vi "__Alicat SD_Test.vi"() -> ()   [LabVIEW 2017]
uses:
  __Alicat SD_ReadingCluster.ctl
  __Alicat SD_Hardware_Module.ctl
panel:
  in  "Used ?":bool=TRUE
  out "Timeout":bool
  in  "CambiarAdd":bool
  out "ParsedReading":T1={"ID"="", "Pressure"=13.55, "Temperature"=28.56, "Volumetric"=-1.9, "Mass"=-1.7, "SetPoint"=250.0, "Gas"=""} {"SetPoint" format="%.2f"; "Mass" format="%.2f"; "Volumetric" format="%.2f"; "Temperature" format="%.2f"; "Pressure" format="%.2f"}
  out "SetPoint (64000=FullScale)":i32=32000 min=0 max=64000 step=1
  in  "Address":string="A"
  out "Cycle":i32
  out "error out":errorcluster
  in  "SetFlow":bool
  in  "VISA resource name":refnum<visa-resource-name>
  in  "stop":bool
  # "Alicat mfc test routine"
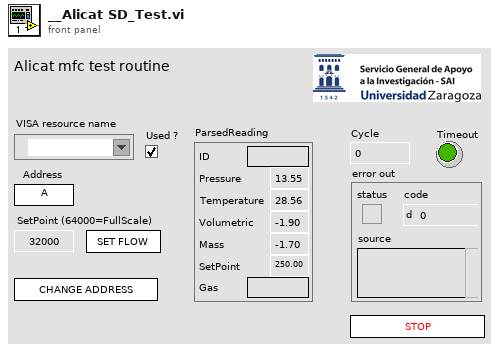
[diagram p1: front panel]
types:
  T1 = typedef "__Alicat SD_ReadingCluster.ctl" = cluster{"ID":string, "Pressure":sgl, "Temperature":sgl, "Volumetric":sgl, "Mass":sgl, "SetPoint":sgl, "Gas":string}
  T2 = typedef "__Alicat SD_Hardware_Module.ctl" = enum16{"Initialize", "Send Setpoint", "Read Data", "Change Address", "Shutdown"}
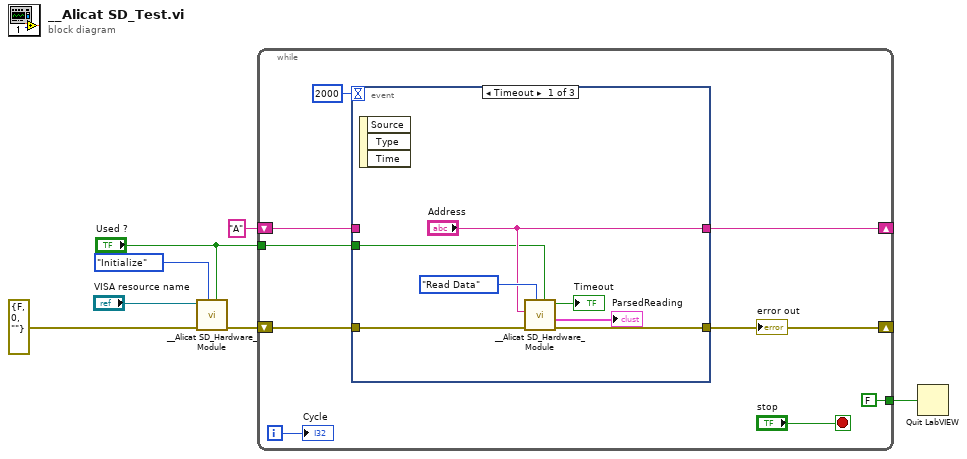
[diagram p0: block diagram]
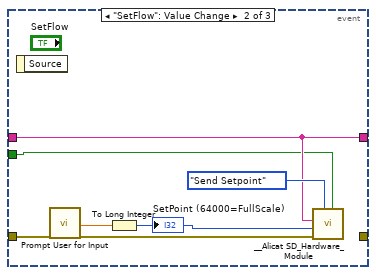
[diagram p2: hidden frame]
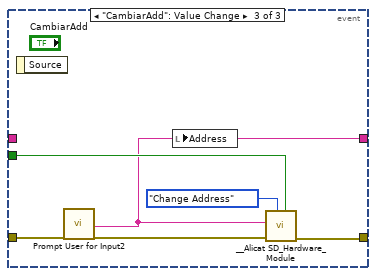
[diagram p3: hidden frame]
diagram:
  n1 = call "__Alicat SD_Hardware_Module.vi"("Used ?"="Used ?", "Command"=__Alicat_SD_Hardware_Module."Initialize", "error in (no error)"=errorcluster {"status"=FALSE, "code"=0, "source"=""}, "VISA resource name"="VISA resource name") -> ("error out"=w7:errorcluster)  [unwired: 4 in, 3 out]
  n2 = while {
    shift-right: [w12] -> _
    shift-left: w7 -> [w13]
    tunnel: [FALSE ("stop")] -> w4
    shift-right: [w10] -> _
    shift-left: "A" ("Address") -> [w11]
    tunnel: "Used ?" -> [w9]
    i -> [w16]
    stop <- "stop" stop-if-true
    n3 = event shown="[0] Timeout" {
      selector: _ -> [_ _ _]
      dyn-events: _ -> [_ _ _]
      timeout: 2000 -> [_ _ _]
      tunnel: w13 -> [w20 w28 w34]
      tunnel: [w19 _ w35] -> w12
      tunnel: w11 -> [_ w29 _]
      tunnel: ["Address" w29 w31] -> w10
      tunnel: w9 -> [w17 w24 w32]
      event Timeout {
        n4 = event-data() -> ()  [unwired: 1 in, 3 out]
        n5 = call "__Alicat SD_Hardware_Module.vi"("Used ?"=w17, "Command"=__Alicat_SD_Hardware_Module."Read Data", "error in (no error)"=w20, "Address"="Address") -> ("error out"=w19:errorcluster, "ParsedReading"=→"ParsedReading":T1, "Timeout"=→"Timeout":bool)  [unwired: 4 in, 1 out]
      }
      event "SetFlow": Value Change {
        n6 = event-data() -> ()  [unwired: 1 in, 1 out]
        n7 = call "Prompt User for Input"("error in (no error)"=w28) -> ("Setpoint"=w26:dbl, "error out"=w27:errorcluster)  [unwired: 16 in, 1 out]
        n8 = To Long Integer(number=w26) -> (32bit integer=w25:i32)
        "SetPoint (64000=FullScale)" <- w25
        n9 = call "__Alicat SD_Hardware_Module.vi"("Used ?"=w24, "Command"=__Alicat_SD_Hardware_Module."Send Setpoint", "error in (no error)"=w27, "SetPoint (64000=FullScale)"=w25, "Address"=w29) -> ()  [unwired: 3 in, 4 out]
      }
      event "CambiarAdd": Value Change {
        n10 = event-data() -> ()  [unwired: 1 in, 1 out]
        n11 = call "Prompt User for Input2"("error in (no error)"=w34) -> ("Setpoint"=w31:string, "error out"=w33:errorcluster)  [unwired: 16 in, 1 out]
        n12 = local write "Address"(w31) -> ()
        n13 = call "__Alicat SD_Hardware_Module.vi"("Used ?"=w32, "Command"=__Alicat_SD_Hardware_Module."Change Address", "error in (no error)"=w33, "Address"=w31) -> ("error out"=w35:errorcluster)  [unwired: 4 in, 3 out]
      }
    }
    "error out" <- w12
    "Cycle" <- w16
  }
  n14 = Quit LabVIEW(quit? (T)=w4) -> ()
